vi "Material.Build Scheme Array.vi"(11 "schemes":T2={"light"={"primary"="", "surfaceTint"="", "onPrimary"="", "primaryContainer"="0", "onPrimaryContainer"="0", "secondary"="0", "onSecondary"="0", "secondaryContainer"="0", "onSecondaryContainer"="0", "tertiary"="0", "onTertiary"="0", "tertiaryContainer"="0", "onTertiaryContainer"="0", "error"="0", "onError"="0", "errorContainer"="0", "onErrorContainer"="0", "background"="0", "onBackground"="0", "surface"="0", "onSurface"="0", "surfaceVariant"="0", "onSurfaceVariant"="0", "outline"="0", "outlineVariant"="0", "shadow"="0", "scrim"="0", "inverseSurface"="0", "inverseOnSurface"="0", "inversePrimary"="", "primaryFixed"="0", "onPrimaryFixed"="0", "primaryFixedDim"="0", "onPrimaryFixedVariant"="0", "secondaryFixed"="0", "onSecondaryFixed"="0", "secondaryFixedDim"="0", "onSecondaryFixedVariant"="0", "tertiaryFixed"="0", "onTertiaryFixed"="0", "tertiaryFixedDim"="0", "onTertiaryFixedVariant"="0", "surfaceDim"="0", "surfaceBright"="0", "surfaceContainerLowest"="0", "surfaceContainerLow"="0", "surfaceContainer"="0", "surfaceContainerHigh"="0", "surfaceContainerHighest"="0"}, "light-medium-contrast"={"primary"="", "surfaceTint"="", "onPrimary"="", "primaryContainer"="0", "onPrimaryContainer"="0", "secondary"="0", "onSecondary"="0", "secondaryContainer"="0", "onSecondaryContainer"="0", "tertiary"="0", "onTertiary"="0", "tertiaryContainer"="0", "onTertiaryContainer"="0", "error"="0", "onError"="0", "errorContainer"="0", "onErrorContainer"="0", "background"="0", "onBackground"="0", "surface"="0", "onSurface"="0", "surfaceVariant"="0", "onSurfaceVariant"="0", "outline"="0", "outlineVariant"="0", "shadow"="0", "scrim"="0", "inverseSurface"="0", "inverseOnSurface"="0", "inversePrimary"="", "primaryFixed"="0", "onPrimaryFixed"="0", "primaryFixedDim"="0", "onPrimaryFixedVariant"="0", "secondaryFixed"="0", "onSecondaryFixed"="0", "secondaryFixedDim"="0", "onSecondaryFixedVariant"="0", "tertiaryFixed"="0", "onTertiaryFixed"="0", "tertiaryFixedDim"="0", "onTertiaryFixedVariant"="0", "surfaceDim"="0", "surfaceBright"="0", "surfaceContainerLowest"="0", "surfaceContainerLow"="0", "surfaceContainer"="0", "surfaceContainerHigh"="0", "surfaceContainerHighest"="0"}, "light-high-contrast"={"primary"="", "surfaceTint"="", "onPrimary"="", "primaryContainer"="0", "onPrimaryContainer"="0", "secondary"="0", "onSecondary"="0", "secondaryContainer"="0", "onSecondaryContainer"="0", "tertiary"="0", "onTertiary"="0", "tertiaryContainer"="0", "onTertiaryContainer"="0", "error"="0", "onError"="0", "errorContainer"="0", "onErrorContainer"="0", "background"="0", "onBackground"="0", "surface"="0", "onSurface"="0", "surfaceVariant"="0", "onSurfaceVariant"="0", "outline"="0", "outlineVariant"="0", "shadow"="0", "scrim"="0", "inverseSurface"="0", "inverseOnSurface"="0", "inversePrimary"="", "primaryFixed"="0", "onPrimaryFixed"="0", "primaryFixedDim"="0", "onPrimaryFixedVariant"="0", "secondaryFixed"="0", "onSecondaryFixed"="0", "secondaryFixedDim"="0", "onSecondaryFixedVariant"="0", "tertiaryFixed"="0", "onTertiaryFixed"="0", "tertiaryFixedDim"="0", "onTertiaryFixedVariant"="0", "surfaceDim"="0", "surfaceBright"="0", "surfaceContainerLowest"="0", "surfaceContainerLow"="0", "surfaceContainer"="0", "surfaceContainerHigh"="0", "surfaceContainerHighest"="0"}, "dark"={"primary"="", "surfaceTint"="", "onPrimary"="", "primaryContainer"="0", "onPrimaryContainer"="0", "secondary"="0", "onSecondary"="0", "secondaryContainer"="0", "onSecondaryContainer"="0", "tertiary"="0", "onTertiary"="0", "tertiaryContainer"="0", "onTertiaryContainer"="0", "error"="0", "onError"="0", "errorContainer"="0", "onErrorContainer"="0", "background"="0", "onBackground"="0", "surface"="0", "onSurface"="0", "surfaceVariant"="0", "onSurfaceVariant"="0", "outline"="0", "outlineVariant"="0", "shadow"="0", "scrim"="0", "inverseSurface"="0", "inverseOnSurface"="0", "inversePrimary"="", "primaryFixed"="0", "onPrimaryFixed"="0", "primaryFixedDim"="0", "onPrimaryFixedVariant"="0", "secondaryFixed"="0", "onSecondaryFixed"="0", "secondaryFixedDim"="0", "onSecondaryFixedVariant"="0", "tertiaryFixed"="0", "onTertiaryFixed"="0", "tertiaryFixedDim"="0", "onTertiaryFixedVariant"="0", "surfaceDim"="0", "surfaceBright"="0", "surfaceContainerLowest"="0", "surfaceContainerLow"="0", "surfaceContainer"="0", "surfaceContainerHigh"="0", "surfaceContainerHighest"="0"}, "dark-medium-contrast"={"primary"="", "surfaceTint"="", "onPrimary"="", "primaryContainer"="0", "onPrimaryContainer"="0", "secondary"="0", "onSecondary"="0", "secondaryContainer"="0", "onSecondaryContainer"="0", "tertiary"="0", "onTertiary"="0", "tertiaryContainer"="0", "onTertiaryContainer"="0", "error"="0", "onError"="0", "errorContainer"="0", "onErrorContainer"="0", "background"="0", "onBackground"="0", "surface"="0", "onSurface"="0", "surfaceVariant"="0", "onSurfaceVariant"="0", "outline"="0", "outlineVariant"="0", "shadow"="0", "scrim"="0", "inverseSurface"="0", "inverseOnSurface"="0", "inversePrimary"="", "primaryFixed"="0", "onPrimaryFixed"="0", "primaryFixedDim"="0", "onPrimaryFixedVariant"="0", "secondaryFixed"="0", "onSecondaryFixed"="0", "secondaryFixedDim"="0", "onSecondaryFixedVariant"="0", "tertiaryFixed"="0", "onTertiaryFixed"="0", "tertiaryFixedDim"="0", "onTertiaryFixedVariant"="0", "surfaceDim"="0", "surfaceBright"="0", "surfaceContainerLowest"="0", "surfaceContainerLow"="0", "surfaceContainer"="0", "surfaceContainerHigh"="0", "surfaceContainerHighest"="0"}, "dark-high-contrast"={"primary"="", "surfaceTint"="", "onPrimary"="", "primaryContainer"="0", "onPrimaryContainer"="0", "secondary"="0", "onSecondary"="0", "secondaryContainer"="0", "onSecondaryContainer"="0", "tertiary"="0", "onTertiary"="0", "tertiaryContainer"="0", "onTertiaryContainer"="0", "error"="0", "onError"="0", "errorContainer"="0", "onErrorContainer"="0", "background"="0", "onBackground"="0", "surface"="0", "onSurface"="0", "surfaceVariant"="0", "onSurfaceVariant"="0", "outline"="0", "outlineVariant"="0", "shadow"="0", "scrim"="0", "inverseSurface"="0", "inverseOnSurface"="0", "inversePrimary"="", "primaryFixed"="0", "onPrimaryFixed"="0", "primaryFixedDim"="0", "onPrimaryFixedVariant"="0", "secondaryFixed"="0", "onSecondaryFixed"="0", "secondaryFixedDim"="0", "onSecondaryFixedVariant"="0", "tertiaryFixed"="0", "onTertiaryFixed"="0", "tertiaryFixedDim"="0", "onTertiaryFixedVariant"="0", "surfaceDim"="0", "surfaceBright"="0", "surfaceContainerLowest"="0", "surfaceContainerLow"="0", "surfaceContainer"="0", "surfaceContainerHigh"="0", "surfaceContainerHighest"="0"}}) -> (2 "scheme":refnum<class "Material-Scheme.lvclass">[](array[class]))   [LabVIEW 2021, in "TSC Material Theme.lvlib" / "Material-Scheme.lvclass"]
doc: "build the array of scheme objects from the original data\n\n<b>Code Developed By:</b>\nTechnology Service Corporation\nwww.tsc.com/atcs\n\nDeveloper:\nDaniel Coons"
uses:
  Material-Scheme.lvclass
  _Material Theme SubVIs/material json scheme.ctl
  Material-Scheme.lvclass/Material-Scheme.ctl
  TSC Material Theme.lvlib
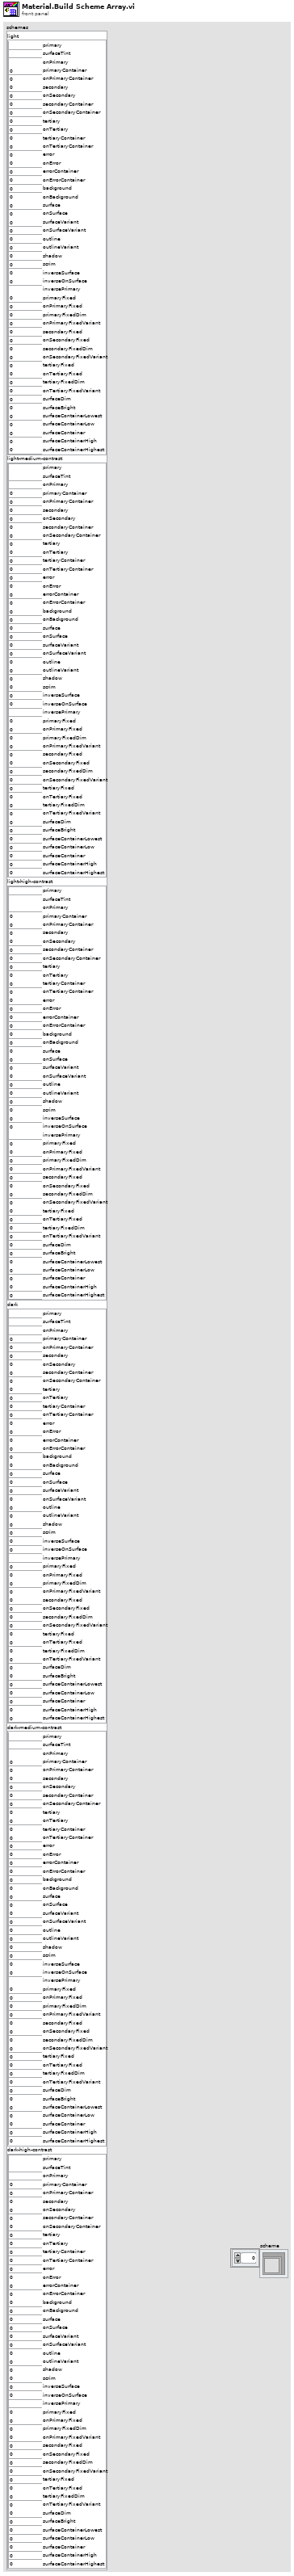
[diagram p1: front panel]
types:
  T1 = typedef "material json scheme.ctl" = cluster{"primary":string, "surfaceTint":string, "onPrimary":string, "primaryContainer":string, "onPrimaryContainer":string, "secondary":string, "onSecondary":string, "secondaryContainer":string, "onSecondaryContainer":string, "tertiary":string, "onTertiary":string, "tertiaryContainer":string, "onTertiaryContainer":string, "error":string, "onError":string, "errorContainer":string, "onErrorContainer":string, "background":string, "onBackground":string, "surface":string, "onSurface":string, "surfaceVariant":string, "onSurfaceVariant":string, "outline":string, "outlineVariant":string, "shadow":string, "scrim":string, "inverseSurface":string, "inverseOnSurface":string, "inversePrimary":string, "primaryFixed":string, "onPrimaryFixed":string, "primaryFixedDim":string, "onPrimaryFixedVariant":string, "secondaryFixed":string, "onSecondaryFixed":string, "secondaryFixedDim":string, "onSecondaryFixedVariant":string, "tertiaryFixed":string, "onTertiaryFixed":string, "tertiaryFixedDim":string, "onTertiaryFixedVariant":string, "surfaceDim":string, "surfaceBright":string, "surfaceContainerLowest":string, "surfaceContainerLow":string, "surfaceContainer":string, "surfaceContainerHigh":string, "surfaceContainerHighest":string}
  T2 = cluster{"light":T1, "light-medium-contrast":T1, "light-high-contrast":T1, "dark":T1, "dark-medium-contrast":T1, "dark-high-contrast":T1}
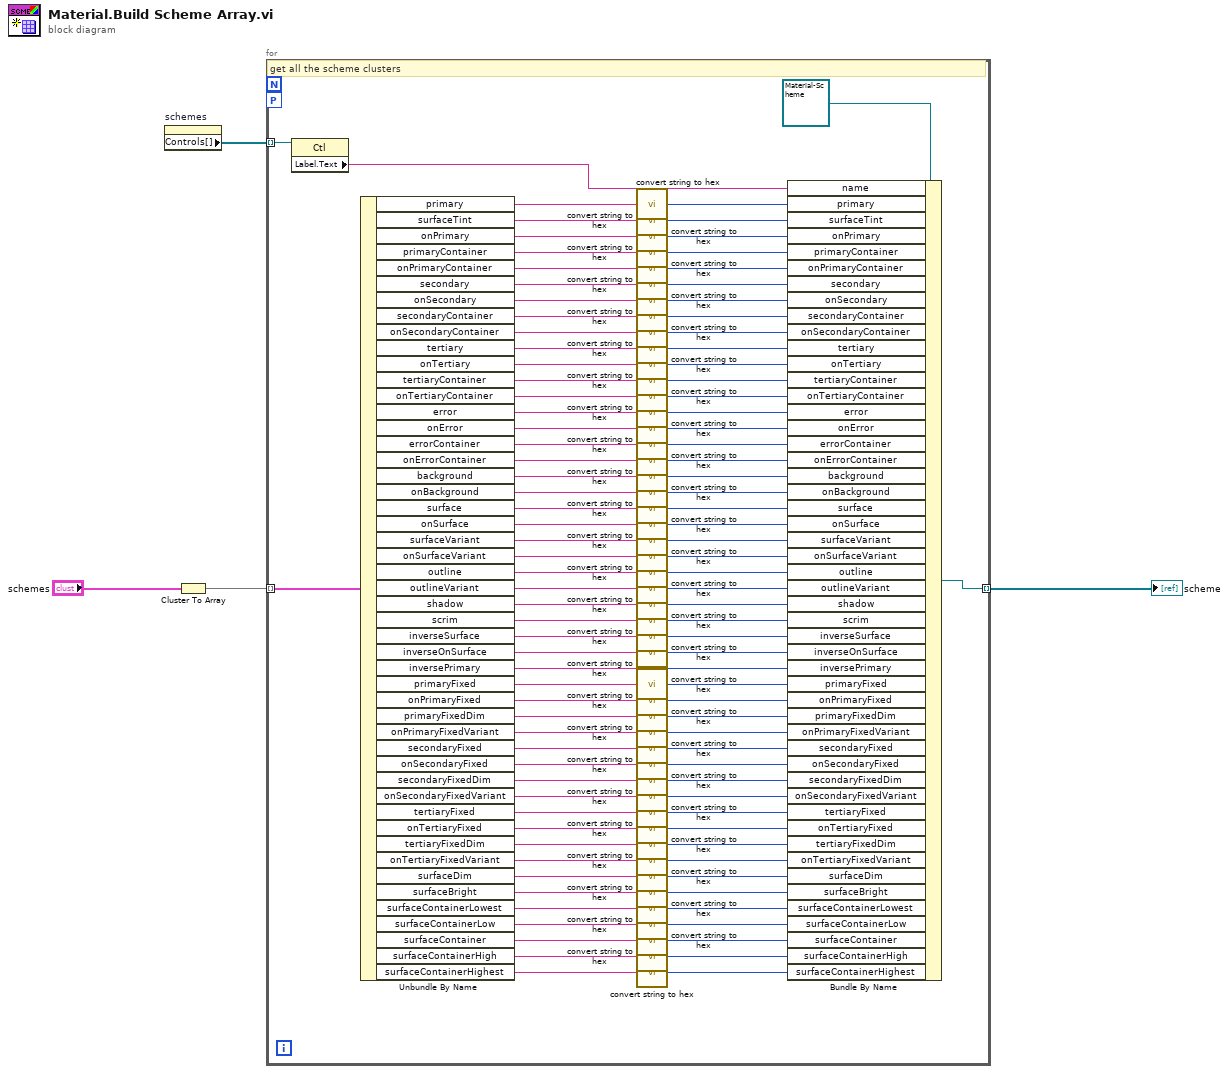
[diagram p0: block diagram]
diagram:
  n1 = property on="schemes" class="Clust (strict)"() -> ("Controls[]"=w1:refnum<vi>[])  [unwired: 2 in, 2 out]
  n2 = Cluster To Array(cluster="schemes") -> (array=w3:T1[])
  n3 = for {
    tunnel: w3 -> [w5] mode=indexing
    tunnel: [w10] -> w4 mode=indexing
    tunnel: w1 -> [w7] mode=indexing
    workers-P: _ -> [_]
    # "get all the scheme clusters"
    n4 = property class="Ctl"(reference=w7) -> ("Label.Text"=w6:string)  [unwired: 1 in, 2 out]
    n5 = Unbundle By Name(w5) -> ("primary"=w106:string, "surfaceTint"=w104:string, "onPrimary"=w103:string, "primaryContainer"=w102:string, "onPrimaryContainer"=w101:string, "secondary"=w100:string, "onSecondary"=w99:string, "secondaryContainer"=w98:string, "onSecondaryContainer"=w97:string, "tertiary"=w96:string, "onTertiary"=w95:string, "tertiaryContainer"=w94:string, "onTertiaryContainer"=w93:string, "error"=w92:string, "onError"=w91:string, "errorContainer"=w90:string, "onErrorContainer"=w89:string, "background"=w88:string, "onBackground"=w87:string, "surface"=w86:string, "onSurface"=w85:string, "surfaceVariant"=w84:string, "onSurfaceVariant"=w83:string, "outline"=w82:string, "outlineVariant"=w81:string, "shadow"=w80:string, "scrim"=w79:string, "inverseSurface"=w78:string, "inverseOnSurface"=w77:string, "inversePrimary"=w9:string, "primaryFixed"=w76:string, "onPrimaryFixed"=w75:string, "primaryFixedDim"=w74:string, "onPrimaryFixedVariant"=w73:string, "secondaryFixed"=w72:string, "onSecondaryFixed"=w71:string, "secondaryFixedDim"=w70:string, "onSecondaryFixedVariant"=w69:string, "tertiaryFixed"=w68:string, "onTertiaryFixed"=w67:string, "tertiaryFixedDim"=w66:string, "onTertiaryFixedVariant"=w65:string, "surfaceDim"=w64:string, "surfaceBright"=w63:string, "surfaceContainerLowest"=w62:string, "surfaceContainerLow"=w61:string, "surfaceContainer"=w60:string, "surfaceContainerHigh"=w59:string, "surfaceContainerHighest"=w11:string)
    n6 = call "convert string to hex.vi"("string"=w106) -> ("hex"=w105:u32)
    n7 = call "convert string to hex.vi"("string"=w104) -> ("hex"=w58:u32)
    n8 = call "convert string to hex.vi"("string"=w103) -> ("hex"=w57:u32)
    n9 = call "convert string to hex.vi"("string"=w102) -> ("hex"=w56:u32)
    n10 = call "convert string to hex.vi"("string"=w101) -> ("hex"=w55:u32)
    n11 = call "convert string to hex.vi"("string"=w100) -> ("hex"=w54:u32)
    n12 = call "convert string to hex.vi"("string"=w99) -> ("hex"=w53:u32)
    n13 = call "convert string to hex.vi"("string"=w98) -> ("hex"=w52:u32)
    n14 = call "convert string to hex.vi"("string"=w97) -> ("hex"=w51:u32)
    n15 = call "convert string to hex.vi"("string"=w96) -> ("hex"=w50:u32)
    n16 = call "convert string to hex.vi"("string"=w95) -> ("hex"=w49:u32)
    n17 = call "convert string to hex.vi"("string"=w94) -> ("hex"=w48:u32)
    n18 = call "convert string to hex.vi"("string"=w93) -> ("hex"=w47:u32)
    n19 = call "convert string to hex.vi"("string"=w92) -> ("hex"=w46:u32)
    n20 = call "convert string to hex.vi"("string"=w91) -> ("hex"=w45:u32)
    n21 = call "convert string to hex.vi"("string"=w90) -> ("hex"=w44:u32)
    n22 = call "convert string to hex.vi"("string"=w89) -> ("hex"=w43:u32)
    n23 = call "convert string to hex.vi"("string"=w88) -> ("hex"=w42:u32)
    n24 = call "convert string to hex.vi"("string"=w87) -> ("hex"=w41:u32)
    n25 = call "convert string to hex.vi"("string"=w86) -> ("hex"=w40:u32)
    n26 = call "convert string to hex.vi"("string"=w85) -> ("hex"=w39:u32)
    n27 = call "convert string to hex.vi"("string"=w84) -> ("hex"=w38:u32)
    n28 = call "convert string to hex.vi"("string"=w83) -> ("hex"=w37:u32)
    n29 = call "convert string to hex.vi"("string"=w82) -> ("hex"=w36:u32)
    n30 = call "convert string to hex.vi"("string"=w81) -> ("hex"=w35:u32)
    n31 = call "convert string to hex.vi"("string"=w80) -> ("hex"=w34:u32)
    n32 = call "convert string to hex.vi"("string"=w79) -> ("hex"=w33:u32)
    n33 = call "convert string to hex.vi"("string"=w78) -> ("hex"=w32:u32)
    n34 = call "convert string to hex.vi"("string"=w77) -> ("hex"=w31:u32)
    n35 = call "convert string to hex.vi"("string"=w9) -> ("hex"=w8:u32)
    n36 = call "convert string to hex.vi"("string"=w76) -> ("hex"=w30:u32)
    n37 = call "convert string to hex.vi"("string"=w75) -> ("hex"=w29:u32)
    n38 = call "convert string to hex.vi"("string"=w74) -> ("hex"=w28:u32)
    n39 = call "convert string to hex.vi"("string"=w73) -> ("hex"=w27:u32)
    n40 = call "convert string to hex.vi"("string"=w72) -> ("hex"=w26:u32)
    n41 = call "convert string to hex.vi"("string"=w71) -> ("hex"=w25:u32)
    n42 = call "convert string to hex.vi"("string"=w70) -> ("hex"=w24:u32)
    n43 = call "convert string to hex.vi"("string"=w69) -> ("hex"=w23:u32)
    n44 = call "convert string to hex.vi"("string"=w68) -> ("hex"=w22:u32)
    n45 = call "convert string to hex.vi"("string"=w67) -> ("hex"=w21:u32)
    n46 = call "convert string to hex.vi"("string"=w66) -> ("hex"=w20:u32)
    n47 = call "convert string to hex.vi"("string"=w65) -> ("hex"=w19:u32)
    n48 = call "convert string to hex.vi"("string"=w64) -> ("hex"=w18:u32)
    n49 = call "convert string to hex.vi"("string"=w63) -> ("hex"=w17:u32)
    n50 = call "convert string to hex.vi"("string"=w62) -> ("hex"=w16:u32)
    n51 = call "convert string to hex.vi"("string"=w61) -> ("hex"=w15:u32)
    n52 = call "convert string to hex.vi"("string"=w60) -> ("hex"=w14:u32)
    n53 = call "convert string to hex.vi"("string"=w59) -> ("hex"=w13:u32)
    n54 = call "convert string to hex.vi"("string"=w11) -> ("hex"=w12:u32)
    n55 = Bundle By Name(cluster=refnum<class "Material-Scheme.lvclass"> refnum ("Material-Scheme.lvclass"), "name"=w6, "primary"=w105, "surfaceTint"=w58, "onPrimary"=w57, "primaryContainer"=w56, "onPrimaryContainer"=w55, "secondary"=w54, "onSecondary"=w53, "secondaryContainer"=w52, "onSecondaryContainer"=w51, "tertiary"=w50, "onTertiary"=w49, "tertiaryContainer"=w48, "onTertiaryContainer"=w47, "error"=w46, "onError"=w45, "errorContainer"=w44, "onErrorContainer"=w43, "background"=w42, "onBackground"=w41, "surface"=w40, "onSurface"=w39, "surfaceVariant"=w38, "onSurfaceVariant"=w37, "outline"=w36, "outlineVariant"=w35, "shadow"=w34, "scrim"=w33, "inverseSurface"=w32, "inverseOnSurface"=w31, "inversePrimary"=w8, "primaryFixed"=w30, "onPrimaryFixed"=w29, "primaryFixedDim"=w28, "onPrimaryFixedVariant"=w27, "secondaryFixed"=w26, "onSecondaryFixed"=w25, "secondaryFixedDim"=w24, "onSecondaryFixedVariant"=w23, "tertiaryFixed"=w22, "onTertiaryFixed"=w21, "tertiaryFixedDim"=w20, "onTertiaryFixedVariant"=w19, "surfaceDim"=w18, "surfaceBright"=w17, "surfaceContainerLowest"=w16, "surfaceContainerLow"=w15, "surfaceContainer"=w14, "surfaceContainerHigh"=w13, "surfaceContainerHighest"=w12) -> (w10:refnum<class "Material-Scheme.lvclass">)
  }
  "scheme" <- w4
